vi "solar_voy_def Import (Header).vi"(10 "DEFAULT_TARGET":string, 11 "HEADER":enum8{"LINC", "CCSDS"}(ring)) -> (2 "TLM_HDR":T1, 3 "CMD_HDR":T1)   [LabVIEW 2018]
doc: "This imports the default LINC and CCSDS headers. \n\nLINC Header:\nU32: HDR_LENGTH\nU16: HDR_ID\nU128: HDR_GUID\n\nVoyager requires the HDR_LENGTH to be a 32 bit size."
uses:
  solar_voy_def_ctl ITEM TYPE.ctl
  type/solar_type Item Type.ctl
  solar_voy_def_ctl ITEM.ctl
  solar_voy_def_ctl HDR.ctl
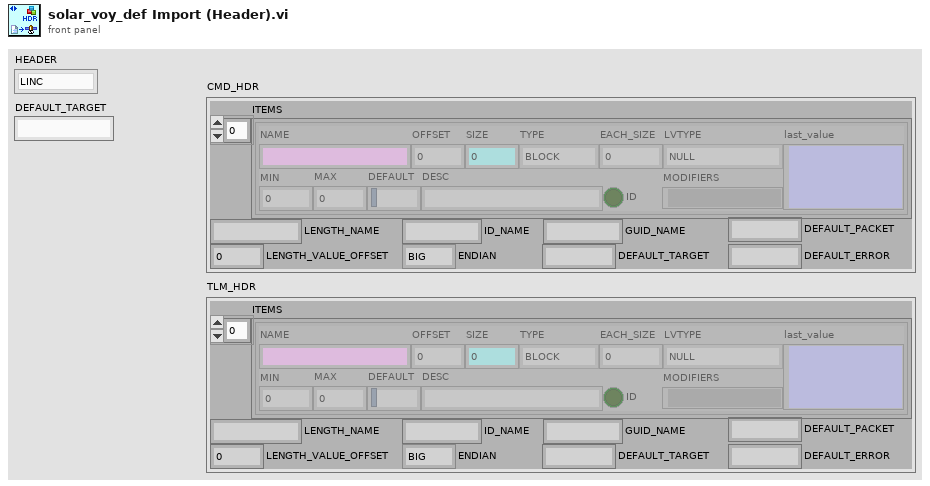
[diagram p1: front panel]
types:
  T1 = typedef "solar_voy_def_ctl HDR.ctl" = cluster{"ITEMS":T2[], "LENGTH_NAME":string, "LENGTH_VALUE_OFFSET":i32, "ID_NAME":string, "ENDIAN":enum8{"BIG", "LITTLE"}, "GUID_NAME":string, "DEFAULT_TARGET":string, "DEFAULT_PACKET":string, "DEFAULT_ERROR":string}
  T2 = typedef "solar_voy_def_ctl ITEM.ctl" = cluster{"NAME":string, "OFFSET":i32, "SIZE":i32, "TYPE":T3, "EACH_SIZE":i32, "LVTYPE":T4, "MIN":dbl, "MAX":dbl, "DEFAULT":string, "DESC":string, "ID":bool, "MODIFIERS":variant, "last_value":variant}
  T3 = typedef "solar_voy_def_ctl ITEM TYPE.ctl" = enum8{"BLOCK", "INT", "UINT", "FLOAT", "STRING"}
  T4 = typedef "solar_type Item Type.ctl" = enum16{"NULL", "UNKNOWN", "CLUSTER", "I8", "I16", "I32", "I64", "U8", "U16", "U32", "U64", "U8_ENUM", "U16_ENUM", "U32_ENUM", "SGL", "DBL", "BOOLEAN", "STRING", "PATH", "VISA", "TAG", "TIME", "I8_1D", "I16_1D", "I32_1D", "I64_1D", "U8_1D", "U16_1D", "U32_1D", "U64_1D", "U8_ENUM_1D", "U16_ENUM_1D", "U32_ENUM_1D", "SGL_1D", "DBL_1D", "BOOLEAN_1D", "STRING_1D", "PATH_1D", "VISA_1D", "TAG_1D", "TIME_1D", "I8_2D", "I16_2D", "I32_2D", "I64_2D", "U8_2D", "U16_2D", "U32_2D", "U64_2D", "U8_ENUM_2D", "U16_ENUM_2D", "U32_ENUM_2D", "SGL_2D", "DBL_2D", "BOOLEAN_2D", "STRING_2D", "PATH_2D", "VISA_2D", "TAG_2D", "TIME_2D"}
  T5 = cluster{"HDR_LENGTH":u32, "HDR_ID,id":u16, "HDR_GUID,t=block,b=128":string}
  T6 = cluster{"HDR_TYPE,b=5":u8, "HDR_ID,b=11,id":u16, "HDR_FLAGS,b=2":u16, "HDR_COUNT,b=14":u16, "HDR_LENGTH":u16, "HDR_DAY":u16, "HDR_MSEC":u32, "HDR_USEC":u16}
  T7 = cluster{"HDR_TYPE,b=5":u8, "HDR_ID,b=11,id":u16, "HDR_FLAGS,b=2":u16, "HDR_COUNT,b=14":u16, "HDR_LENGTH":u16}
  T8 = typedef "solar_voy_def_ctl PACKET.ctl" = cluster{"PACKET_ID":T9, "ENDIAN":enum8{"BIG", "LITTLE"}, "DESC":string, "HZRD":bool, "ITEMS":T2[], "NoExport":bool, "last_time":timestamp, "last_count":u32, "last_data":string}
  T9 = typedef "solar_voy_def_ctl PACKET_ID.ctl" = cluster{"ID":u16, "CMD":enum8{"CMD", "TLM"}, "TARGET":string, "PACKET":string}
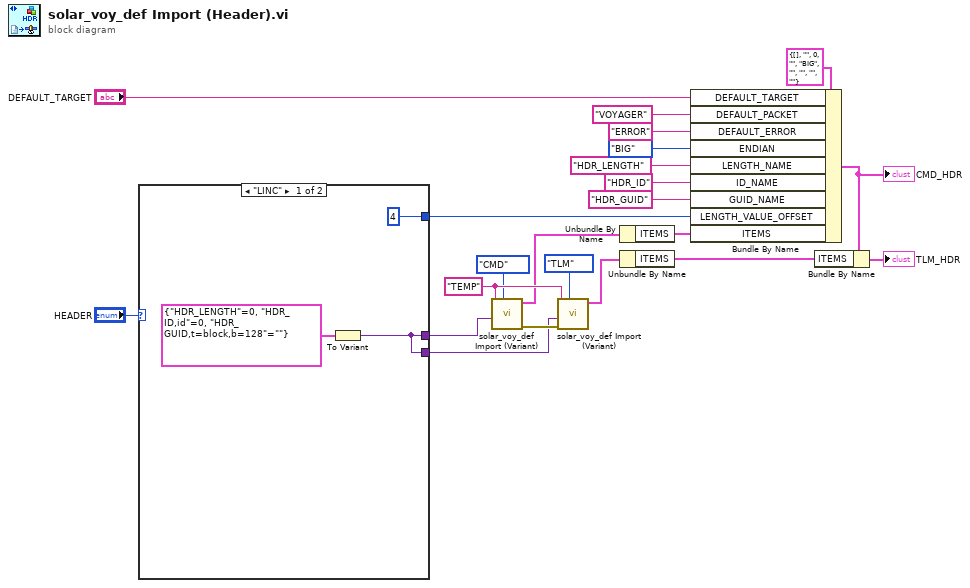
[diagram p0: block diagram]
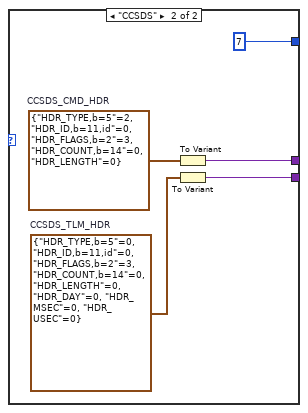
[diagram p2: hidden frame]
diagram:
  w21 = "TEMP" ("TARGET")
  n1 = case shown="\"LINC\"" "HEADER" {
    tunnel: [w24 w29] -> w15
    tunnel: [w24 w27] -> w14
    tunnel: [4 ("LENGTH_VALUE_OFFSET") 7 ("LENGTH_VALUE_OFFSET")] -> w2
    frame "LINC" {
      n2 = To Variant(anything=T5 {"HDR_LENGTH"=0, "HDR_ID,id"=0, "HDR_GUID,t=block,b=128"=""} ("LINC_HDR")) -> (Variant=w24:variant)
    }
    frame "CCSDS" {
      w28 = T6 {"HDR_TYPE,b=5"=0, "HDR_ID,b=11,id"=0, "HDR_FLAGS,b=2"=3, "HDR_COUNT,b=14"=0, "HDR_LENGTH"=0, "HDR_DAY"=0, "HDR_MSEC"=0, "HDR_USEC"=0}  # CCSDS_TLM_HDR
      w30 = T7 {"HDR_TYPE,b=5"=2, "HDR_ID,b=11,id"=0, "HDR_FLAGS,b=2"=3, "HDR_COUNT,b=14"=0, "HDR_LENGTH"=0}  # CCSDS_CMD_HDR
      n3 = To Variant(anything=w30) -> (Variant=w29:variant)
      n4 = To Variant(anything=w28) -> (Variant=w27:variant)
    }
  }
  n5 = call "solar_voy_def Import (Variant).vi"("CMD"=enum8{"CMD", "TLM"}."CMD", "Variant"=w15, "TARGET"=w21) -> ("error out"=w18:errorcluster, "PACKET"=w19:T8)  [unwired: 7 in]
  n6 = call "solar_voy_def Import (Variant).vi"("CMD"=enum8{"CMD", "TLM"}."TLM", "error in (no error)"=w18, "Variant"=w14, "TARGET"=w21) -> ("PACKET"=w20:T8)  [unwired: 6 in, 1 out]
  n7 = Unbundle By Name(w19) -> ("ITEMS"=w13:T2[])
  n8 = Unbundle By Name(w20) -> ("ITEMS"=w10:T2[])
  n9 = Bundle By Name(cluster=T1 {"ITEMS"=[], "LENGTH_NAME"="", "LENGTH_VALUE_OFFSET"=0, "ID_NAME"="", "ENDIAN"=enum."BIG", "GUID_NAME"="", "DEFAULT_TARGET"="", "DEFAULT_PACKET"="", "DEFAULT_ERROR"=""} ("CMD_HDR"), "DEFAULT_TARGET"="DEFAULT_TARGET", "DEFAULT_PACKET"="VOYAGER", "DEFAULT_ERROR"="ERROR", "ENDIAN"=enum8{"BIG", "LITTLE"}."BIG", "LENGTH_NAME"="HDR_LENGTH", "ID_NAME"="HDR_ID", "GUID_NAME"="HDR_GUID", "LENGTH_VALUE_OFFSET"=w2, "ITEMS"=w13) -> (w3:T1)
  "CMD_HDR" <- w3
  n10 = Bundle By Name(cluster=w3, "ITEMS"=w10) -> (→"TLM_HDR":T1)
